vi "Send Message.vi"(8 "error in (no error)":errorcluster, 10 "String in":string, 11 "TCP Writer in":refnum<class "TCP Writer.lvclass">) -> (0 "error out":errorcluster, 3 "TCP Writer out":refnum<class "TCP Writer.lvclass">)   [LabVIEW 2026, in "TALOS.lvlib" / "TCP Writer.lvlib" / "TCP Writer.lvclass"]
uses:
  TCP Writer.lvclass
  C:/LabVIEW Code/TALOS/talos/Father of all uServices/Father of all uServices/Father of all uServices.lvclass
  TCP Writer.lvclass/TCP Writer.ctl
  Father of all uServices/Father of all uServices/Father of all uServices.lvclass/Father of all uServices.ctl
  Ancestor/Ancestor/Ancestor.lvclass/Ancestor.ctl
  TCP Writer Consumer Case Selector.ctl
  Father of all uServices/Father of all uServices Messages/Consumer Msg/Consumer Msg.lvclass/Consumer Msg.ctl
  Father of all uServices/Father of all uServices/Children Methods/Update GUI.vi
  FGV/Error Memory/Get Error Description.vi
  Support VIs/Get PC name.vi
  Ancestor/Ancestor/Read ID.vi
  Support VIs/Get Class Name.vi
  <vilib>/Utility/error.llb/Clear Errors.vi
  Father of all uServices/Father of all uServices Messages/Consumer Msg/Send Consumer.vi
  FGV/Error Memory/Error Memory Core.vi
  <vilib>/AdvancedString/Delimited String to 1D String Array.vi
  <vilib>/AdvancedString/Delimited String to 1D String Array (string).vi
  Support VIs/Circus Root Path.vi
  FGV/Error Memory/Error Crt Lvl checker.vi
  FGV/Error Memory/Error Memory Core.vi/40c8088d-b597-4017-91af-faa98e00292e.vi
  FGV/Error Memory/Error Memory Core.vi/d4a3ab98-063c-4e44-b43d-fbdcfe6c2be2.vi
  Father of all uServices/Father of all uServices/Father of all uServices.lvclass
  C:/LabVIEW Code/TALOS/builds/Actor Framework PPL/Actor Framework.lvlibp/1abvi3w/vi.lib/ActorFramework/Actor/Actor.lvclass
  Support VIs/Global Constants.vi
  Father of all uServices/Father of all uServices/Children Methods/Get GUI Item Value - String.vi
  Father of all uServices/Father of all uServices/Multiline string updater.vi
  Support VIs/Global Memory.vi
  <vilib>/Utility/LVClass/Get LV Class Name.vi
  Support VIs/Is in Packed Library.vi
  Support VIs/TALOS Root path.vi
  Support VIs/Read CSV worksheet.vi
  <vilib>/Utility/error.llb/General Error Handler.vi
  Support VIs/Error Log.vi
  builds/Actor Framework PPL/Actor Framework.lvlibp/1abvi3w/vi.lib/ActorFramework/Actor/Read Self Enqueuer.vi
  <userlib>/_OpenG.lib/lvdata/lvdata.llb/Get Strings from Enum__ogtk.vi
  builds/Actor Framework PPL/Actor Framework.lvlibp/1abvi3w/vi.lib/ActorFramework/Message Enqueuer/Enqueue.vi
  Ancestor/Ancestor/Ancestor.lvclass
  <vilib>/Comparison/Equal/Equal Functor/Equal Functor.lvclass
  Father of all uServices/Father of all uServices Messages/Consumer Msg/Consumer Msg.lvclass
  TALOS.lvlib
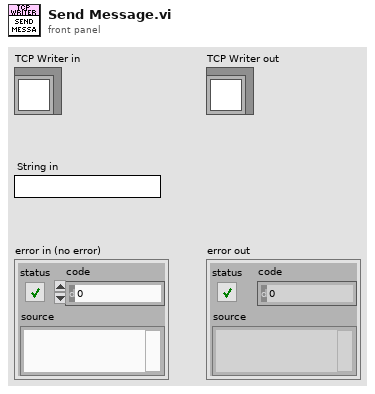
[diagram p1: front panel]
types:
  T1 = typedef "TALOS.lvlib/TCP Writer.lvlib/TCP Writer.lvclass/TCP Writer Consumer Case Selector.ctl" = enum16{"Send message", "Idle", "Check Connection", "Open connection", "Set Client ID"}
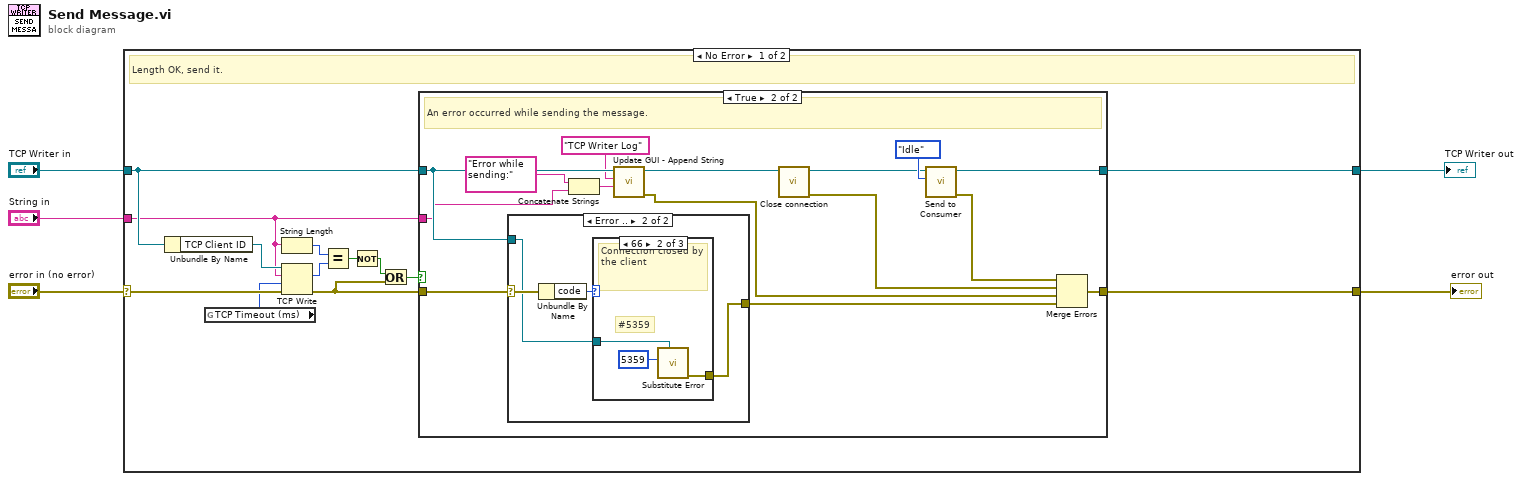
[diagram p0: block diagram]
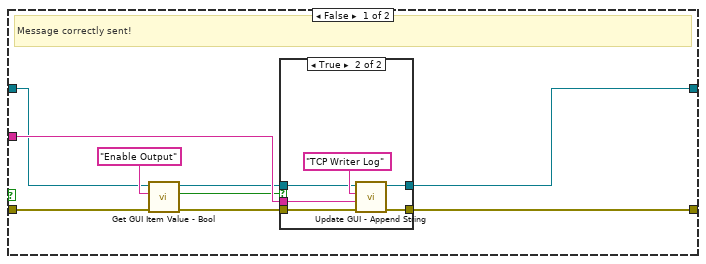
[diagram p2: hidden frame]
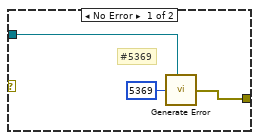
[diagram p4: hidden frame]
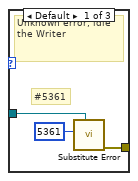
[diagram p5: hidden frame]
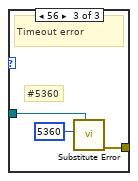
[diagram p6: hidden frame]
diagram:
  n1 = case shown="No Error" "error in (no error)" {
    selector: "error in (no error)" -> [w16 w68]
    tunnel: [w18 w68] -> w1
    tunnel: "TCP Writer in" -> [w15 w67]
    tunnel: "String in" -> [w6 _]
    tunnel: [w17 w67] -> w2
    frame No Error {
      # "Length OK, send it."
      n2 = Unbundle By Name(w15) -> ("TCP Client ID"=w14:refnum<k5>)
      n3 = global read "Global Constants.vi" "TCP Timeout (ms)"() -> (w13:i32)
      n4 = String Length(string=w6) -> (length=w12:i32)
      n5 = TCP Write(connection ID=w14, data in=w6, error in (no error)=w16, 9:w13) -> (bytes written=w11:i32, error out=w7:errorcluster)  [unwired: 1 out]
      n6 = Equal?(x=w12, y=w11) -> (x = y?=w10:bool)
      n7 = Not(x=w10) -> (.not. x?=w8:bool)
      n8 = Or(x=w8, y=w7) -> (x .or. y?=w9:bool)
      n9 = case shown="True" w9 {
        tunnel: w15 -> [w20 w50]
        tunnel: [w25 w47] -> w18
        tunnel: [w27 w37] -> w17
        tunnel: w7 -> [w23 w45]
        tunnel: w6 -> [w26 w41]
        frame False {
          # "Message correctly sent!"
          n10 = call "Get GUI Item Value - Bool.vi"("error in (no error)"=w23, "FP Item Name"="Enable Output" ("Parameter Name"), "uService Template in"=w20) -> ("error out"=w22:errorcluster, "Value"=w21:bool, "uService Template out"=w19:refnum<class "TCP Writer.lvclass">)  [unwired: 6 in]
          n11 = case shown="True" w21 {
            tunnel: w22 -> [w29 w35]
            tunnel: [w29 w34] -> w25
            tunnel: w26 -> [_ w33]
            tunnel: [w28 w31] -> w27
            tunnel: w19 -> [w28 w30]
            frame False {
            }
            frame True {
              n12 = call "Update GUI - Append String.vi"("error in (no error)"=w35, "String"=w33, "GUI Item Name"="TCP Writer Log", "Father of all uServices in"=w30) -> ("error out"=w34:errorcluster, "Father of all uServices out"=w31:refnum<class "TCP Writer.lvclass">)  [unwired: 6 in]
            }
          }
        }
        frame True {
          # "An error occurred while sending the message."
          n13 = case shown="Error .." w45 {
            selector: w45 -> [_ w55]
            tunnel: [w53 w56] -> w46
            tunnel: w50 -> [w52 w54]
            frame No Error {
              # "#5369"
              n14 = call "Generate Error.vi"("Class"=w52, "Error Code"=5369) -> ("error out"=w53:errorcluster)  [unwired: 5 in]
            }
            frame Error {
              n15 = Unbundle By Name(w55) -> ("code"=w57:i32)
              n16 = case shown="66" w57 {
                tunnel: [w59 w63 w65] -> w56
                tunnel: w54 -> [w58 w61 w64]
                frame Default {
                  # "#5361"
                  # "Unknown error, idle the Writer"
                  n17 = call "Substitute Error.vi"("LabVIEW Object"=w58, "Error Code"=5361) -> ("error out"=w59:errorcluster)  [unwired: 9 in]
                }
                frame 66 {
                  # "#5359"
                  # "Connection closed by the client"
                  n18 = call "Substitute Error.vi"("LabVIEW Object"=w61, "Error Code"=5359) -> ("error out"=w63:errorcluster)  [unwired: 9 in]
                }
                frame 56 {
                  # "#5360"
                  # "Timeout error"
                  n19 = call "Substitute Error.vi"("LabVIEW Object"=w64, "Error Code"=5360) -> ("error out"=w65:errorcluster)  [unwired: 9 in]
                }
              }
            }
          }
          n20 = Concatenate Strings("Error while sending:" ("GUI Item Name"), w41) -> (w40:string)
          n21 = call "Update GUI - Append String.vi"("String"=w40, "GUI Item Name"="TCP Writer Log", "Father of all uServices in"=w50) -> ("error out"=w43:errorcluster, "Father of all uServices out"=w39:refnum<class "TCP Writer.lvclass">)  [unwired: 7 in]
          n22 = call-dynamic "Close connection.vi"("TCP Writer in"=w39) -> ("error out"=w36:errorcluster, "TCP Writer out"=w38:refnum<class "TCP Writer.lvclass">)  [unwired: 9 in]
          n23 = call "Send to Consumer.vi"("Case ID"=TCP_Writer_Consumer_Case_Selector."Idle" ("TCP Listener Consumer Case Selector"), "uService Template in"=w38) -> ("error out"=w49:errorcluster, "uService Template out"=w37:refnum<class "TCP Writer.lvclass">)  [unwired: 8 in]
          n24 = Merge Errors(w49, w36, w43, w46) -> (w47:errorcluster)
        }
      }
    }
    frame Error {
      # "DO not kill the connection: something went wrong with the part generating the message, not the TCP connection itself."
      # "Something went wrong: just let the error go out."
    }
  }
  "TCP Writer out" <- w2
  "error out" <- w1
